vi "Set Event Data.vi"(8 "error in (no error)":errorcluster, 10 "Event Data JSON":string, 11 "BroadcastCustomEvent in":refnum<class "BroadcastCustomEvent.lvclass">) -> (0 "error out":errorcluster, 3 "BroadcastCustomEvent out":refnum<class "BroadcastCustomEvent.lvclass">)   [LabVIEW 2020, in "obs-websocket.lvlib" / "BroadcastCustomEvent.lvclass"]
uses:
  BroadcastCustomEvent.lvclass
  BroadcastCustomEvent.lvclass/BroadcastCustomEvent.ctl
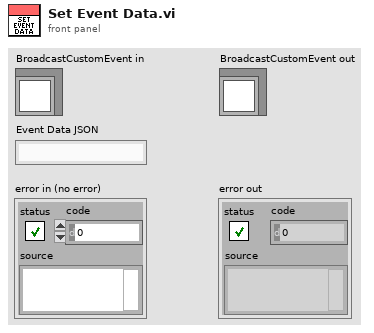
[diagram p1: front panel]
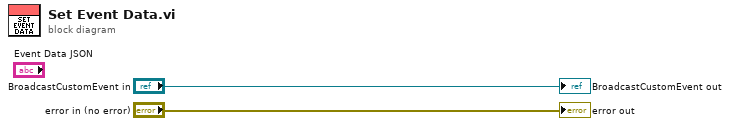
[diagram p0: block diagram]
diagram:
  "error out" <- "error in (no error)"
  "BroadcastCustomEvent out" <- "BroadcastCustomEvent in"
